vi "Set Cooler Power Status.vi"(8 "error in (no error)":errorcluster, 11 "CCDCamera in":refnum<class "Real Camera.lvclass">) -> (0 "error out":errorcluster, 3 "CCDCamera out":refnum<class "Real Camera.lvclass">)   [LabVIEW 2018, in "Real Camera.lvclass"]
doc: "Turn the cooler on or off"
uses:
  Real Camera.lvclass
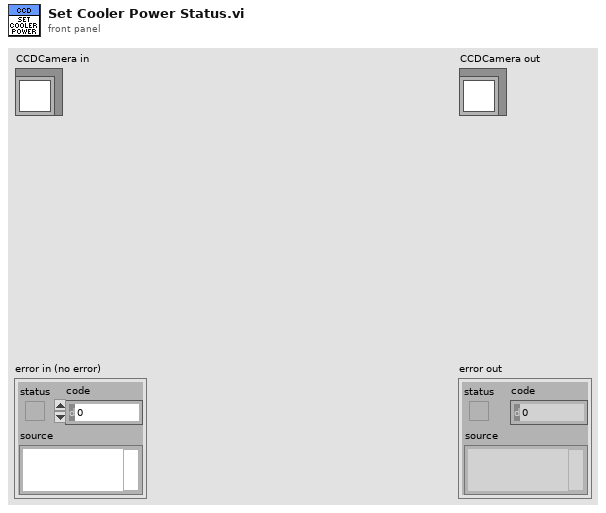
[diagram p1: front panel]
types:
  T1 = cluster{"COOLER_POWER_STATUS":u16, "TEMP":i32, "EXPTIME":dbl, "#FRAMES":u32}
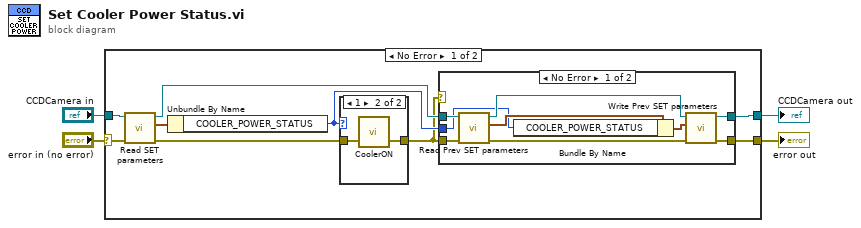
[diagram p0: block diagram]
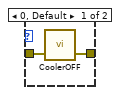
[diagram p3: hidden frame]
diagram:
  n1 = case shown="No Error" "error in (no error)" {
    selector: "error in (no error)" -> [w12 w29]
    tunnel: "CCDCamera in" -> [w13 w30]
    tunnel: [w9 w30] -> w2
    tunnel: [w10 w29] -> w1
    frame No Error {
      n2 = call-dynamic "Read SET parameters.vi"("error in (no error)"=w12, "Simulated_CCD_Camera in"=w13) -> ("error out"=w5:errorcluster, "New SET parameters"=w11:T1, "Simulated_CCD_Camera out"=w7:refnum<class "Real Camera.lvclass">)  [unwired: 7 in]
      n3 = Unbundle By Name(w11) -> ("COOLER_POWER_STATUS"=w8:u16)
      n4 = case shown="1" w8 {
        tunnel: [w26 w28] -> w6
        tunnel: w5 -> [w25 w27]
        frame 0, Default {
          n5 = call <userlib>:"CoolerOFF.vi"("error in (no error)"=w25) -> ("error out"=w26:errorcluster)  [unwired: 1 in, 1 out]
        }
        frame 1 {
          n6 = call <userlib>:"CoolerON.vi"("error in (no error)"=w27) -> ("error out"=w28:errorcluster)  [unwired: 1 in, 1 out]
        }
      }
      n7 = case shown="No Error" w6 {
        tunnel: [w22 w24] -> w9
        tunnel: [w21 w23] -> w10
        tunnel: w7 -> [w17 w24]
        tunnel: w6 -> [w18 w23]
        tunnel: w8 -> [w14 _]
        frame No Error {
          n8 = call-dynamic "Read Prev SET parameters.vi"("error in (no error)"=w18, "Simulated_CCD_Camera in"=w17) -> ("error out"=w19:errorcluster, "Prev SET parameters"=w16:T1, "Simulated_CCD_Camera out"=w20:refnum<class "Real Camera.lvclass">)  [unwired: 7 in]
          n9 = Bundle By Name(cluster=w16, "COOLER_POWER_STATUS"=w14) -> (w15:T1)
          n10 = call-dynamic "Write Prev SET parameters.vi"("error in (no error)"=w19, "Prev SET parameters"=w15, "Simulated_CCD_Camera in"=w20) -> ("error out"=w21:errorcluster, "Simulated_CCD_Camera out"=w22:refnum<class "Real Camera.lvclass">)  [unwired: 7 in]
        }
        frame Error {
        }
      }
    }
    frame Error {
    }
  }
  "error out" <- w1
  "CCDCamera out" <- w2
